vi "reboot.vi"(9 "id":u8, 10 "protocol_version":i32, 11 "port_num":i32) -> ()   [LabVIEW 2021, in "dxl_x86_c.lvlib"]
doc: "#undef reboot\n#define reboot rebootDXL\n#endif\n\n#define BROADCAST_ID 0xFE #define MAX_ID 0xFC \n\n#define DXL_MAKEWORD(a, b) ((uint16_t)(((uint8_t)(((uint64_t)(a)) & 0xff)) | ((uint16_t)((uint8_t)(((uint64_t)(b)) & 0xff))) << 8))\n#define DXL_MAKEDWORD(a, b) ((uint32_t)(((uint16_t)(((uint64_t)(a)) & 0xffff)) | ((uint32_t)((uint16_t)(((uint64_t)(b)) & 0xffff))) << 16))\n#define DXL_LOWORD(l) ((uint16_t)(((uint64_t)(l)) & 0xffff))\n#define DXL_HIWORD(l) ((uint16_t)((((uint64_t)(l)) >> 16) & 0xffff))\n#define DXL_LOBYTE(w) ((uint8_t)(((uint64_t)(w)) & 0xff))\n#define DXL_HIBYTE(w) ((uint8_t)((((uint64_t)(w)) >> 8) & 0xff))\n\n\n#define INST_PING 1\n#define INST_READ 2\n#define INST_WRITE 3\n#define INST_REG_WRITE 4\n#define INST_ACTION 5\n#define INST_FACTORY_RESET 6\n#define INST_SYNC_WRITE 131 #define INST_BULK_READ 146 #define INST_REBOOT 8\n#define INST_CLEAR 16 #define INST_STATUS 85 #define INST_SYNC_READ 130 #define INST_FAST_SYNC_READ 138 #define INST_BULK_WRITE 147 \n#define COMM_SUCCESS 0 #define COMM_PORT_BUSY -1000 #define COMM_TX_FAIL -1001 #define COMM_RX_FAIL -1002 #define COMM_TX_ERROR -2000 #define COMM_RX_WAITING -3000 #define COMM_RX_TIMEOUT -3001 #define COMM_RX_CORRUPT -3002 #define COMM_NOT_AVAILABLE -9000 \ntypedef struct\n{\n uint8_t *data_write;"
uses:
  dxl_x86_c.lvlib
  dxl_x86_c.dll
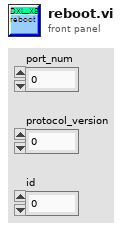
[diagram p1: front panel]
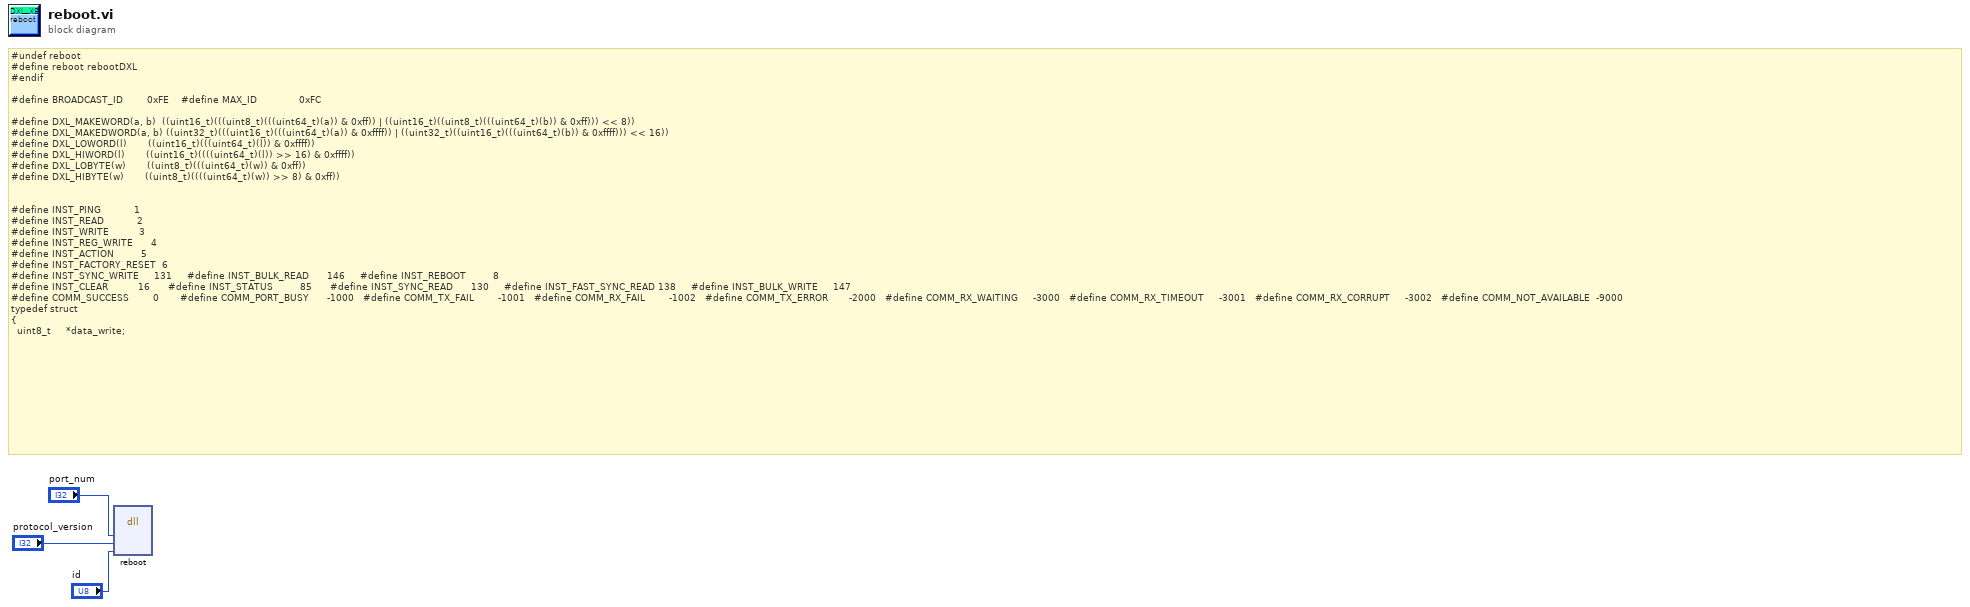
[diagram p0: block diagram]
diagram:
  # "#undef reboot\n#define reboot rebootDXL\n#endif\n\n#define BROADCAST_ID        0xFE    #define MAX_ID              0xFC    \n\n#define DXL_MAKEWORD(a, b)  ((uint16_t)(((uint8_t)(((uint64_t)(a)) & 0xff)) | ((uint16_t)((uint8_t)(((uint64_t)(b)) & 0xff))) << 8))\n#define DXL_MAKEDWORD(a, b) ((uint32_t)(((uint16_t)(((uint64_t)(a)) & 0xffff)) | ((uint32_t)((uint16_t)(((uint64_t)(b)) & 0xffff))) << 16))\n#define DXL_LOWORD(l)       ((uint16_t)(((uint64_t)(l)) & 0xffff))\n#define DXL_HIWORD(l)       ((uint16_t)((((uint64_t)(l)) >> 16) & 0xffff))\n#define DXL_LOBYTE(w)       ((uint8_t)(((uint64_t)(w)) & 0xff))\n#define DXL_HIBYTE(w)       ((uint8_t)((((uint64_t)(w)) >> 8) & 0xff))\n\n\n#define INST_PING           1\n#define INST_READ           2\n#define INST_WRITE          3\n#define INST_REG_WRITE      4\n#define INST_ACTION         5\n#define INST_FACTORY_RESET  6\n#define INST_SYNC_WRITE     131     #define INST_BULK_READ      146     #define INST_REBOOT         8\n#define INST_CLEAR          16      #define INST_STATUS         85      #define INST_SYNC_READ      130     #define INST_FAST_SYNC_READ 138     #define INST_BULK_WRITE     147     \n#define COMM_SUCCESS        0       #define COMM_PORT_BUSY      -1000   #define COMM_TX_FAIL        -1001   #define COMM_RX_FAIL        -1002   #define COMM_TX_ERROR       -2000   #define COMM_RX_WAITING     -3000   #define COMM_RX_TIMEOUT     -3001   #define COMM_RX_CORRUPT     -3002   #define COMM_NOT_AVAILABLE  -9000   \ntypedef struct\n{\n  uint8_t     *data_write;"
  n1 = dll-call lib="C:/Users/ashek/Desktop/ashekim/ws/DynamixelSDK/labview/labview/dxl_x86_c.*" fn="reboot"("port_num"="port_num", "protocol_version"="protocol_version", "id"="id") -> ()  [unwired: 7 in, 2 out]
